vi "Creator.vi"(9 "Priority?":bool, 10 "Msg Strategy":refnum<class "Msg Strategy.lvclass">, 11 "Base jettl in":refnum<class "Base jettl.lvclass">) -> (3 "Base jettl out":refnum<class "Base jettl.lvclass">)   [LabVIEW 2021, in "jettl.lvlib" / "Base jettl.lvclass"]
uses:
  Base jettl.lvclass
  Base jettl.lvclass/Base jettl.ctl
  Sender/Relation.ctl
  Sender/Sender.lvlib
  Sender/Sender/Sender.lvclass
  Msg Strategy/Msg Strategy.lvclass
  Addresses Strategy/Addresses Strategy/Addresses Strategy.lvclass
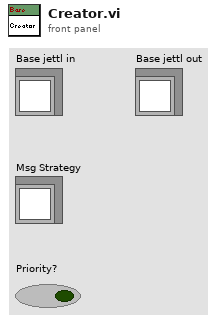
[diagram p1: front panel]
types:
  T1 = typedef "jettl.lvlib/Sender.lvlib/Relation.ctl" = enum16{"Self", "Creator", "Created"}
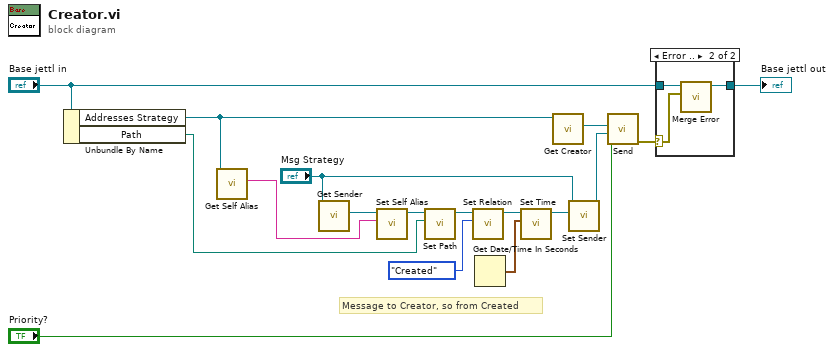
[diagram p0: block diagram]
diagram:
  # "Message to Creator, so from Created"
  n1 = Unbundle By Name("Base jettl in") -> ("Addresses Strategy"=w11:refnum<class "Addresses Strategy.lvclass">, "Path"=w1:path)
  n2 = call-dynamic "Get Self Alias.vi"("Addresses Strategy in"=w11) -> ("Self Alias"=w4:string)  [unwired: 10 in]
  n3 = call-dynamic "Get Sender.vi"("Msg Strategy in"="Msg Strategy") -> ("Sender"=w9:refnum<class "Sender.lvclass">)  [unwired: 10 in]
  n4 = call-dynamic "Set Self Alias.vi"("Self Alias"=w4, "Sender in"=w9) -> ("Sender out"=w8:refnum<class "Sender.lvclass">)  [unwired: 9 in]
  n5 = call-dynamic "Set Path.vi"("Path"=w1, "Sender in"=w8) -> ("Sender out"=w7:refnum<class "Sender.lvclass">)  [unwired: 9 in]
  n6 = call-dynamic "Set Relation.vi"("Relation"=Relation."Created", "Sender in"=w7) -> ("Sender out"=w6:refnum<class "Sender.lvclass">)  [unwired: 9 in]
  n7 = Get Date/Time In Seconds() -> (seconds since 1Jan1904=w2:timestamp)
  n8 = call-dynamic "Set Time.vi"("Time"=w2, "Sender in"=w6) -> ("Sender out"=w5:refnum<class "Sender.lvclass">)  [unwired: 9 in]
  n9 = call-dynamic "Get Creator.vi"("Addresses Strategy in"=w11) -> ("Creator"=w16:refnum<user-event>)  [unwired: 10 in]
  n10 = call-dynamic "Set Sender.vi"("Sender"=w5, "Msg Strategy in"="Msg Strategy") -> ("Msg Strategy out"=w12:refnum<class "Msg Strategy.lvclass">)  [unwired: 9 in]
  n11 = call "Send.vi"("Priority?"="Priority?", "Msg Strategy"=w12, "Msg Event"=w16) -> ("error out"=w17:errorcluster)  [unwired: 8 in]
  n12 = case shown="Error .." w17 {
    selector: w17 -> [_ w19]
    tunnel: [w18 w21] -> w13
    tunnel: "Base jettl in" -> [w18 w20]
    frame No Error {
    }
    frame Error {
      n13 = call-dynamic "Merge Error.vi"("Error"=w19, "Base jettl in"=w20) -> ("Base jettl out"=w21:refnum<class "Base jettl.lvclass">)  [unwired: 9 in]
    }
  }
  "Base jettl out" <- w13
